vi "PH_Stepmotor_BaseClass.Data String to Axis Settings.vi"(0 "Data String":string) -> (1 "No axis":bool, 2 "Axis Settings":T1={"Sign change"=FALSE, "Width"=0.0, "Calibration"=0.0, "Unit"="Steps", "Motor Type"=enum."Unspecific", "Unit Width"="", "Unit CF"=""})   [LabVIEW 2014, in "PH_Stepmotor_BaseClass.lvlib"]
doc: "This VI converts a string to a specific cluster of Axis settings:\n- Sign Change: 1, t, T, true, TRUE or True is converted to \"true\" (boolean), else: \"false\"\n- Width: a number is vonverted to a double\n- Calibration factor: a number is converted to a double\n- Unit: String\n- Motor Type: Number\n\nWithin the string, the arguments must be seperated by \"::\"."
uses:
  PH_Stepmotor_BaseClass.lvlib
  PH_Stepmotor_BaseClass.Axis Settings.ctl
  PH_Stepmotor_BaseClass.Motor Type.ctl
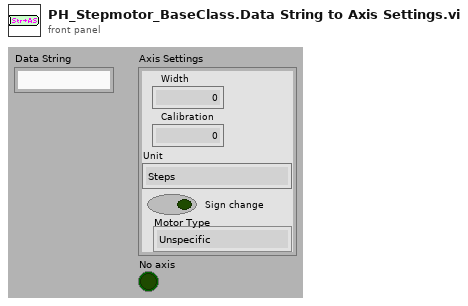
[diagram p1: front panel]
types:
  T1 = typedef "PH_Stepmotor_BaseClass.lvlib/PH_Stepmotor_BaseClass.Axis Settings.ctl" = cluster{"Sign change":bool, "Width":dbl, "Calibration":dbl, "Unit":string, "Motor Type":T2, "Unit Width":string, "Unit CF":string}
  T2 = typedef "PH_Stepmotor_BaseClass.lvlib/PH_Stepmotor_BaseClass.Motor Type.ctl" = enum16{"Unspecific", "OWIS 49.120.2633", "OWIS 49.060.1033", "OWIS 43.040.2558", "Diamond Motion 2200 series", "OWIS 49.120.266B.MV6", "Calorimeter", "Linear Stage 1", "MICOS VT-80", "MICOS VT-80 S", "Standa Rotstage nt0.95A", "PUF RA 320.200", "PUF RA 800.200", "PUF RA 800.400", "PUF RA 400.50", "1324.nn.800.50", "1324.n9c.800.50", "1324.nn.320.200", "1324.nn.400.200", "1324.nn.800.200", "1324.nn.400.50", "1324.8c9c.800.50", "1324.8c9c.400.200"}
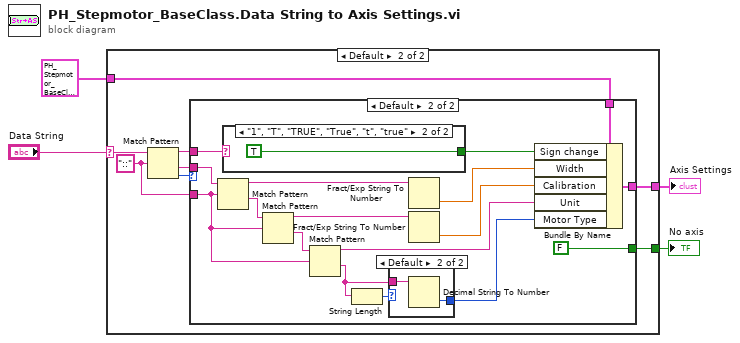
[diagram p0: block diagram]
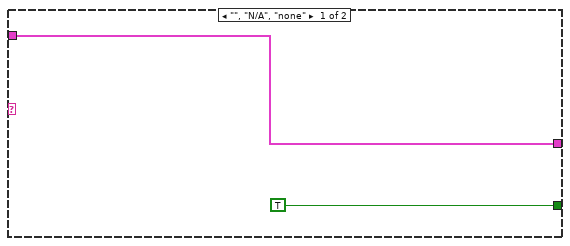
[diagram p2: hidden frame]
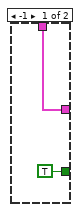
[diagram p3: hidden frame]
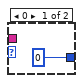
[diagram p4: hidden frame]
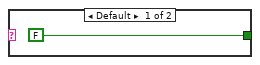
[diagram p5: hidden frame]
diagram:
  n1 = case shown="Default" "Data String" {
    selector: "Data String" -> [_ w9]
    tunnel: T1 {"Sign change"=FALSE, "Width"=0.0, "Calibration"=0.0, "Unit"="Steps", "Motor Type"=enum."Unspecific", "Unit Width"="", "Unit CF"=""} ("Axis Settings") -> [w6 w11]
    tunnel: [w6 w10] -> w3
    tunnel: [TRUE w7] -> w1
    frame "", "N/A", "none" {
    }
    frame Default {
      w12 = "::" ("regular expression")
      n2 = Match Pattern(string=w9, regular expression=w12) -> (before substring=w14:string, after substring=w13:string, offset past match=w8:i32)  [unwired: 1 in, 1 out]
      n3 = case shown="Default" w8 {
        tunnel: w14 -> [_ w31]
        tunnel: w13 -> [_ w29]
        tunnel: w12 -> [_ w27]
        tunnel: w11 -> [w16 w24]
        tunnel: [w16 w23] -> w10
        tunnel: [TRUE FALSE] -> w7
        frame -1 {
        }
        frame Default {
          n4 = Match Pattern(string=w29, regular expression=w27) -> (before substring=w32:string, after substring=w30:string)  [unwired: 1 in, 2 out]
          n5 = case shown="\"1\", \"T\", \"TRUE\", \"True\", \"t\", \"true\"" w31 {
            tunnel: [FALSE TRUE] -> w22
            frame Default {
            }
            frame "1", "T", "TRUE", "True", "t", "true" {
            }
          }
          n6 = Match Pattern(string=w30, regular expression=w27) -> (before substring=w33:string, after substring=w28:string)  [unwired: 1 in, 2 out]
          n7 = Match Pattern(string=w28, regular expression=w27) -> (before substring=w19:string, after substring=w26:string)  [unwired: 1 in, 2 out]
          n8 = String Length(string=w26) -> (length=w25:i32)
          n9 = case shown="Default" w25 {
            tunnel: w26 -> [_ w36]
            tunnel: [0 w35] -> w18
            frame 0 {
            }
            frame Default {
              n10 = Decimal String To Number(string=w36) -> (number=w35:i32)  [unwired: 2 in, 1 out]
            }
          }
          n11 = Fract/Exp String To Number(string=w32) -> (number=w21:dbl)  [unwired: 3 in, 1 out]
          n12 = Fract/Exp String To Number(string=w33) -> (number=w20:dbl)  [unwired: 3 in, 1 out]
          n13 = Bundle By Name(cluster=w24, "Sign change"=w22, "Width"=w21, "Calibration"=w20, "Unit"=w19, "Motor Type"=w18) -> (w23:T1)
        }
      }
    }
  }
  "Axis Settings" <- w3
  "No axis" <- w1
